vi "Interprete message.vi"(8 "error in (no error)":errorcluster, 11 "TCS in":refnum<class "TCS.lvclass">) -> (0 "error out":errorcluster, 3 "TCS out":refnum<class "TCS.lvclass">)   [LabVIEW 2018, in "TCS.lvclass"]
uses:
  TCS.lvclass
  Telemetry/Telemetry.lvclass
  C:/Users/observer/Desktop/Sparc4GUI/SPARC4_GUI/Device/Device.lvclass
panel:
  in  "TCS parameters":T1
  out "error out 2":errorcluster
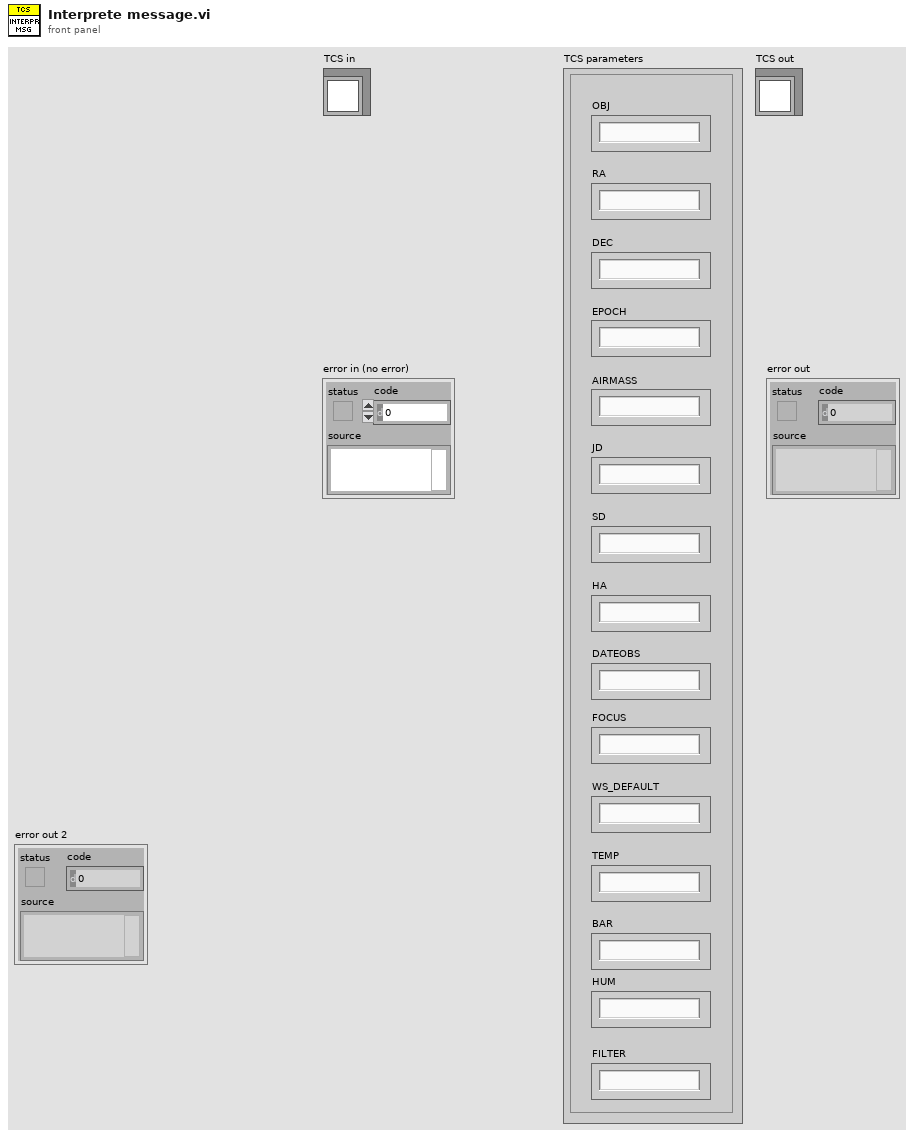
[diagram p1: front panel]
types:
  T1 = cluster{"OBJ":string, "RA":string, "DEC":string, "EPOCH":string, "AIRMASS":string, "JD":string, "SD":string, "HA":string, "DATEOBS":string, "FOCUS":string, "WS_DEFAULT":string, "TEMP":string, "BAR":string, "HUM":string, "FILTER":string}
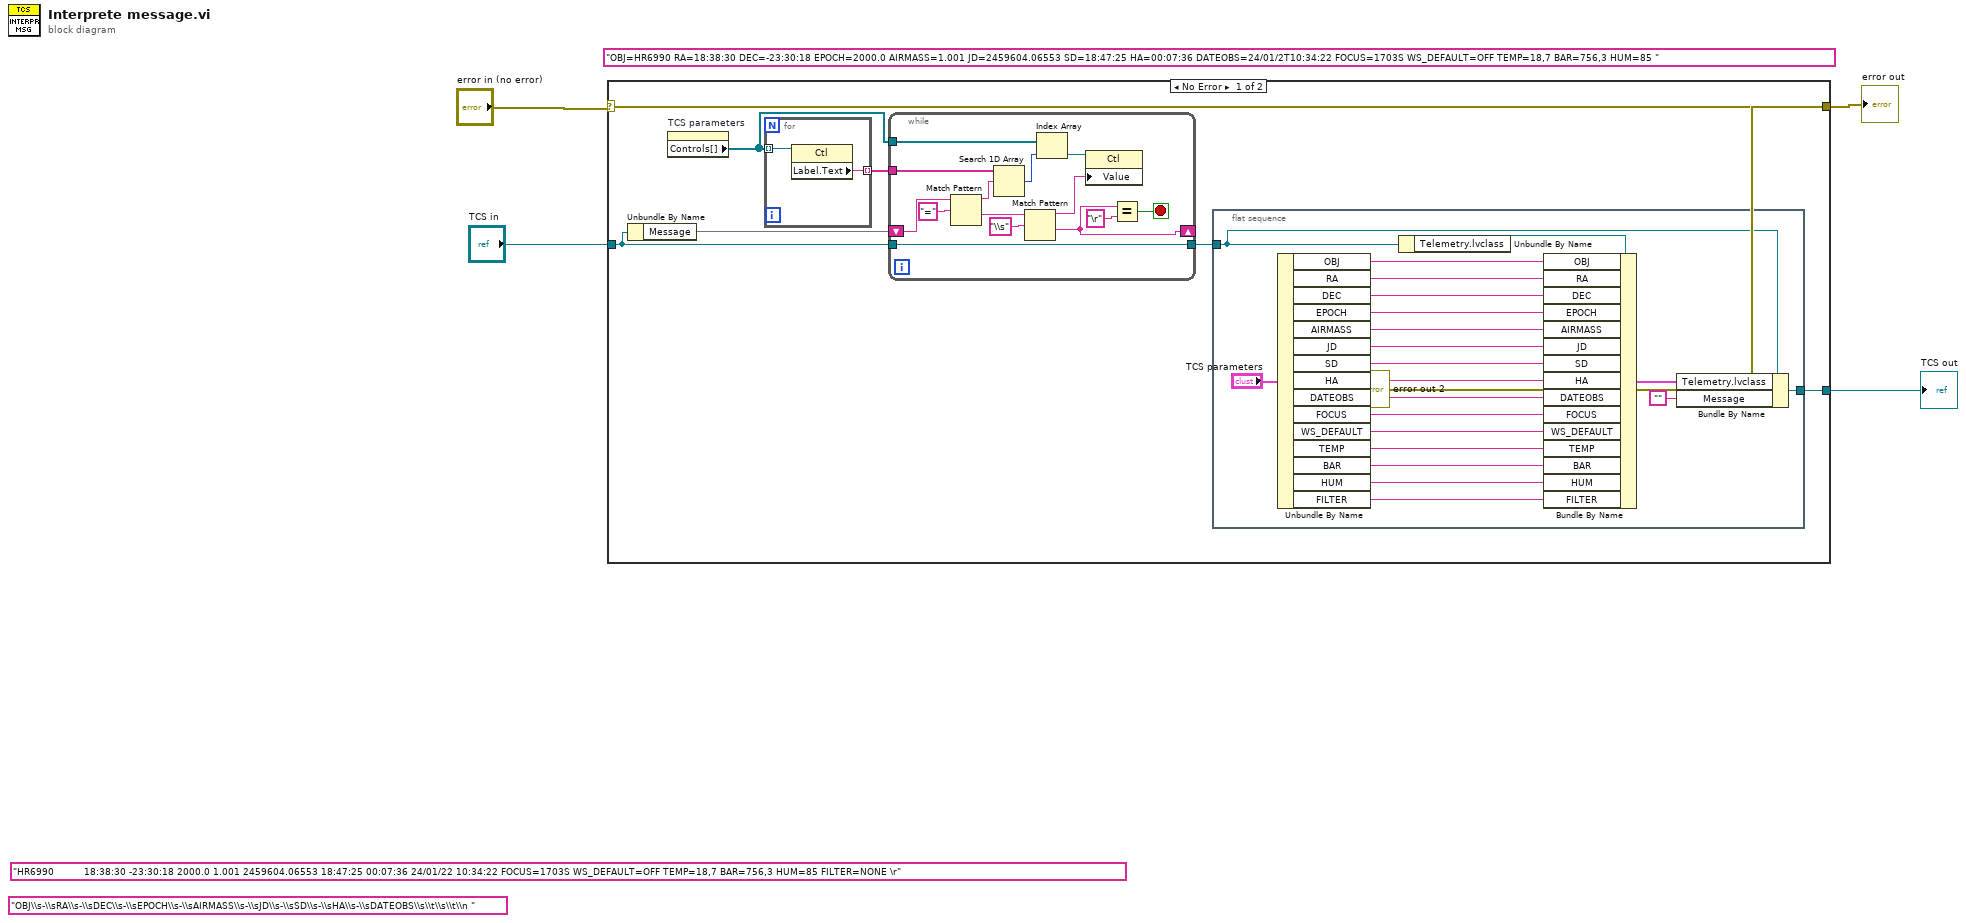
[diagram p0: block diagram]
diagram:
  (unwired) "OBJ=HR6990 RA=18:38:30 DEC=-23:30:18 EPOCH=2000.0 AIRMASS=1.001 JD=2459604.06553 SD=18:47:25 HA=00:07:36 DATEOBS=24/01/2T10:34:22 FOCUS=1703S WS_DEFAULT=OFF TEMP=18,7 BAR=756,3 HUM=85 "
  (unwired) "OBJ\\s-\\sRA\\s-\\sDEC\\s-\\sEPOCH\\s-\\sAIRMASS\\s-\\sJD\\s-\\sSD\\s-\\sHA\\s-\\sDATEOBS\\s\\t\\s\\t\\n "
  (unwired) "HR6990          18:38:30 -23:30:18 2000.0 1.001 2459604.06553 18:47:25 00:07:36 24/01/22 10:34:22 FOCUS=1703S WS_DEFAULT=OFF TEMP=18,7 BAR=756,3 HUM=85 FILTER=NONE \r"
  n1 = case shown="No Error" "error in (no error)" {
    selector: "error in (no error)" -> [w11 w50]
    tunnel: [w11 w50] -> w2
    tunnel: [w6 w49] -> w1
    tunnel: "TCS in" -> [w8 w49]
    frame No Error {
      n2 = Unbundle By Name(w8) -> ("Message"=w5)
      n3 = property on="TCS parameters" class="Clust (strict)"() -> ("Controls[]"=w9:refnum<vi>[])  [unwired: 2 in, 2 out]
      n4 = for {
        tunnel: w9 -> [w34] mode=indexing
        tunnel: [w33] -> w10 mode=indexing
        n5 = property class="Ctl"(reference=w34) -> ("Label.Text"=w33:string)  [unwired: 1 in, 2 out]
      }
      n6 = while {
        shift-right: [w43] -> _
        shift-left: w5 -> [w47]
        tunnel: w8 -> [w36]
        tunnel: w10 -> [w38]
        tunnel: w9 -> [w37]
        tunnel: [w36] -> w7
        stop <- w44 stop-if-true
        n7 = Match Pattern(string=w47, regular expression="=") -> (before substring=w40:string, after substring=w46:string)  [unwired: 1 in, 2 out]
        n8 = Search 1D Array(1D array=w38, element=w40) -> (index of element=w41:i32)  [unwired: 1 in]
        n9 = Match Pattern(string=w46, regular expression="\\s") -> (before substring=w42:string, after substring=w43:string)  [unwired: 1 in, 2 out]
        n10 = Index Array(array=w37, index=w41) -> (element=w39:refnum<vi>)
        n11 = property class="Ctl"(reference=w39, "Value"=w42) -> ()  [unwired: 1 in, 2 out]
        n12 = Equal?(x=w43, y="\r") -> (x = y?=w44:bool)
      }
      n13 = flat-sequence {
        tunnel: w7 -> [w29]
        tunnel: [w32] -> w6
        frame #0 {
          n14 = Unbundle By Name("TCS parameters") -> ("OBJ"=w17:string, "RA"=w18:string, "DEC"=w19:string, "EPOCH"=w12:string, "AIRMASS"=w13:string, "JD"=w14:string, "SD"=w20:string, "HA"=w21:string, "DATEOBS"=w22:string, "FOCUS"=w23:string, "WS_DEFAULT"=w24:string, "TEMP"=w25:string, "BAR"=w26:string, "HUM"=w27:string, "FILTER"=w15:string)
          n15 = Unbundle By Name(w29) -> ("Telemetry.lvclass"=w28:refnum<class "Telemetry.lvclass">)
          n16 = Bundle By Name(cluster=w28, "OBJ"=w17, "RA"=w18, "DEC"=w19, "EPOCH"=w12, "AIRMASS"=w13, "JD"=w14, "SD"=w20, "HA"=w21, "DATEOBS"=w22, "FOCUS"=w23, "WS_DEFAULT"=w24, "TEMP"=w25, "BAR"=w26, "HUM"=w27, "FILTER"=w15) -> (w16:cluster{})
          n17 = Bundle By Name(cluster=w29, "Telemetry.lvclass"=w16, "Message"="") -> (w32:refnum<class "TCS.lvclass">)
        }
      }
    }
    frame Error {
    }
  }
  "error out" <- w2
  "error out 2" <- w2
  "TCS out" <- w1
